vi "EditorThumbnail setLayout.vi"(8 "error in (no error)":errorcluster, 11 "EditorThumbnail in":refnum<class "EditorThumbnail.lvclass">) -> (0 "error out":errorcluster, 3 "EditorThumbnail out":refnum<class "EditorThumbnail.lvclass">)   [LabVIEW 2018, in "EditorThumbnail.lvclass"]
uses:
  EditorThumbnail.lvclass
  <vilib>/Utility/miscctls.llb/LVBoundsTypeDef.ctl
  <vilib>/Utility/miscctls.llb/LVPositionTypeDef.ctl
  EditorThumbnail.lvclass/EditorThumbnail.ctl
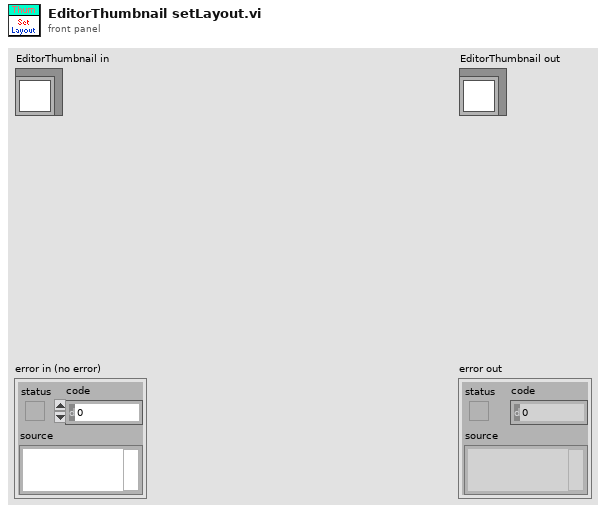
[diagram p1: front panel]
types:
  T1 = typedef "LVPositionTypeDef.ctl" = cluster{"Left":i32, "Top":i32}
  T2 = typedef "LVBoundsTypeDef.ctl" = cluster{"Width":u32, "Height":u32}
  T3 = cluster{"index":u32, "data":cluster{"xdata":dbl[], "ydata":sgl[]}[], "peak":dbl[], "picture":picture}[]
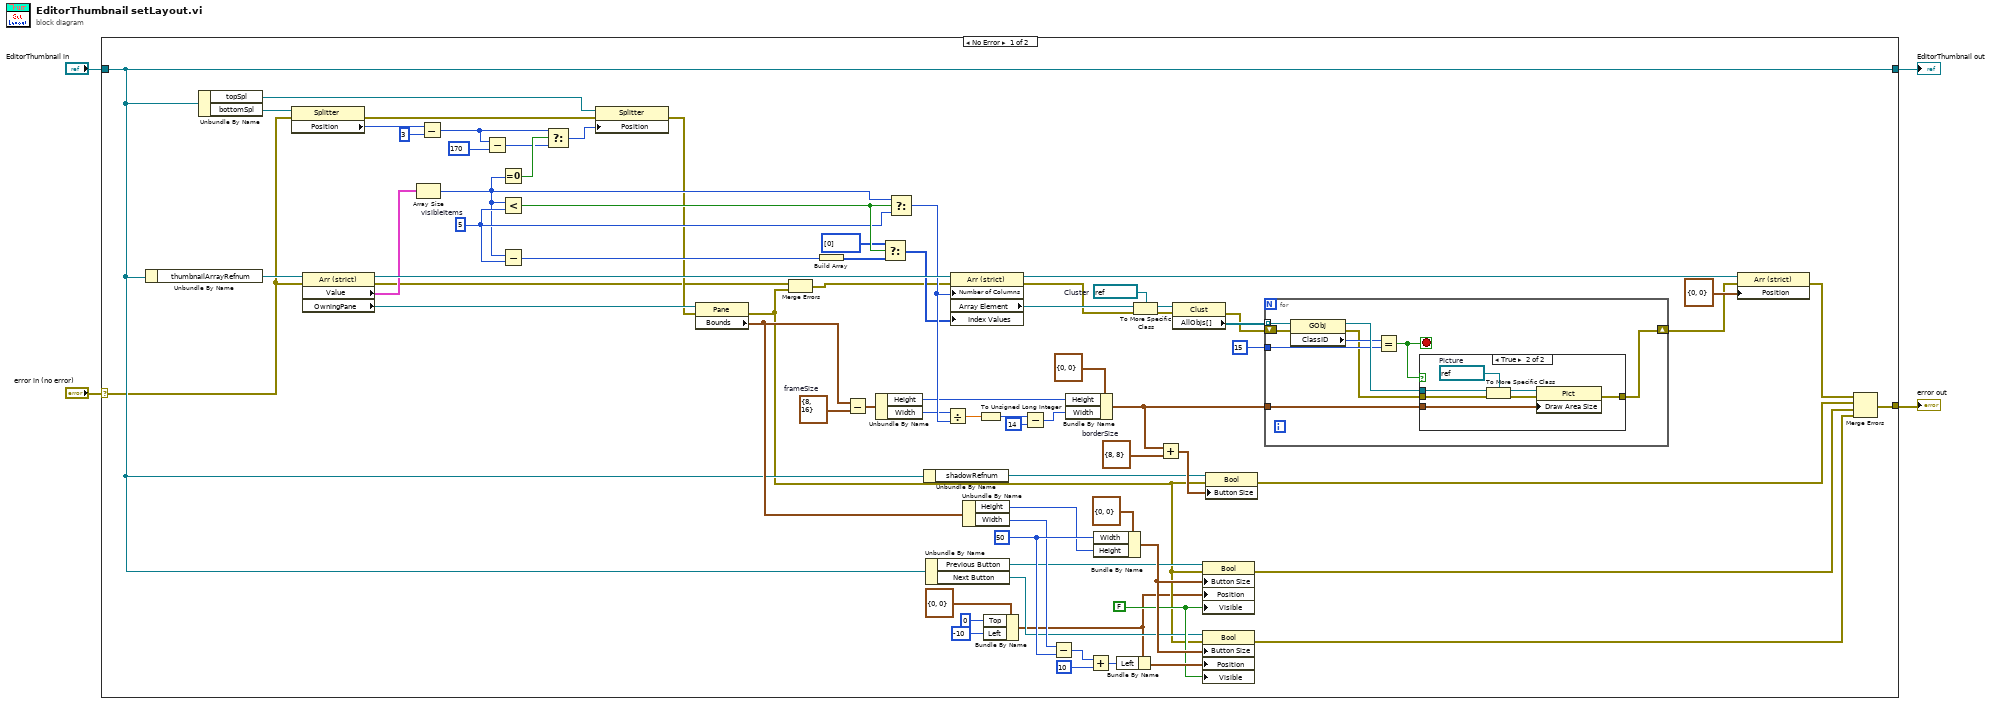
[diagram p0: block diagram]
diagram:
  n1 = case shown="No Error" "error in (no error)" {
    selector: "error in (no error)" -> [w24 w97]
    tunnel: [w49 w97] -> w3
    tunnel: [w26 w96] -> w1
    tunnel: "EditorThumbnail in" -> [w26 w96]
    frame No Error {
      w37 = FALSE ("Visible")
      w40 = u32 50 ("Width")
      w63 = refnum<vi> refnum  # Cluster
      w65 = T2 {"Width"=8, "Height"=8}  # borderSize
      w75 = T2 {"Width"=8, "Height"=16}  # frameSize
      w46 = 5  # visibleItems
      n2 = Unbundle By Name(w26) -> ("thumbnailArrayRefnum"=w78:refnum<vi>)
      n3 = Unbundle By Name(w26) -> ("topSpl"=w15:refnum<vi>, "bottomSpl"=w25:refnum<vi>)
      n4 = property class="Splitter"(reference=w25, error in=w24) -> (error out=w16:errorcluster, "Position"=w21:i32)  [unwired: 1 out]
      n5 = property class="Arr (strict)"(reference=w78, error in=w24) -> (reference out=w76:refnum<vi>, error out=w12:errorcluster, "Value"=w14:T3, "OwningPane"=w77:refnum<vi>)
      n6 = Array Size(array=w14) -> (size(s)=w23:i32)
      n7 = Subtract(x=w21, y=3) -> (x-y=w19:i32)
      n8 = Subtract(x=w19, y=170) -> (x-y=w18:i32)
      n9 = Equal To 0?(x=w23) -> (x = 0?=w20:bool)
      n10 = Less?(x=w23, y=w46) -> (x < y?=w48:bool)
      n11 = Subtract(x=w23, y=w46) -> (x-y=w45:i32)
      n12 = Select(t=w19, s=w20, f=w18) -> (s? t:f=w7:i32)
      n13 = property class="Splitter"(reference=w15, error in=w16, "Position"=w7) -> (error out=w13:errorcluster)  [unwired: 1 out]
      n14 = property class="Pane"(reference=w77, error in=w13) -> (error out=w11:errorcluster, "Bounds"=w36:T2)  [unwired: 1 out]
      n15 = Merge Errors(w12, w11) -> (w10:errorcluster)
      n16 = Build Array(w45) -> (w44:i32[])
      n17 = Subtract(x=w36, y=w75) -> (x-y=w74:T2)
      n18 = Unbundle By Name(w74) -> ("Height"=w68:u32, "Width"=w72:u32)
      n19 = Select(t=u32[] [0] ("Index Values"), s=w48, f=w44) -> (s? t:f=w43:u32[])
      n20 = Select(t=w23, s=w48, f=w46) -> (s? t:f=w73:i32)
      n21 = Unbundle By Name(w26) -> ("shadowRefnum"=w33:refnum<vi>)
      n22 = Unbundle By Name(w26) -> ("Previous Button"=w32:refnum<vi>, "Next Button"=w31:refnum<vi>)
      n23 = Divide(x=w72, y=w73) -> (x/y=w70:dbl)
      n24 = property class="Arr (strict)"(reference=w76, error in=w10, "Number of Columns"=w73, "Index Values"=w43) -> (reference out=w58:refnum<vi>, error out=w56:errorcluster, "Array Element"=w62:refnum<vi>)
      n25 = Unbundle By Name(w36) -> ("Height"=w35:u32, "Width"=w34:u32)
      n26 = To Unsigned Long Integer(number=w70) -> (unsigned 32bit integer=w69:u32)
      n27 = Bundle By Name(cluster=T1 {"Left"=0, "Top"=0} ("Position"), "Top"=0, "Left"=-10) -> (w6:T1)
      n28 = Subtract(x=w69, y=u32 14) -> (x-y=w67:u32)
      n29 = Subtract(x=w34, y=w40) -> (x-y=w38:u32)
      n30 = Bundle By Name(cluster=T2 {"Width"=0, "Height"=0} ("Draw Area Size"), "Height"=w68, "Width"=w67) -> (w59:T2)
      n31 = Add(x=w38, y=u32 10) -> (x+y=w28:u32)
      n32 = Bundle By Name(cluster=T2 {"Width"=0, "Height"=0} ("Button Size"), "Width"=w40, "Height"=w35) -> (w41:T2)
      n33 = Bundle By Name(cluster=w6, "Left"=w28) -> (w39:T1)
      n34 = To More Specific Class(target class=w63, reference=w62, error in=w56) -> (specific class reference=w61:refnum<vi>, error out=w55:errorcluster)
      n35 = Add(x=w59, y=w65) -> (x+y=w64:T2)
      n36 = property class="Clust"(reference=w61, error in=w55) -> (error out=w54:errorcluster, "AllObjs[]"=w60:refnum<vi>[])  [unwired: 1 out]
      n37 = property class="Bool"(reference=w32, error in=w11, "Button Size"=w41, "Position"=w6, "Visible"=w37) -> (error out=w30:errorcluster)  [unwired: 1 out]
      n38 = property class="Bool"(reference=w31, error in=w11, "Button Size"=w41, "Position"=w39, "Visible"=w37) -> (error out=w29:errorcluster)  [unwired: 1 out]
      n39 = property class="Bool"(reference=w33, error in=w11, "Button Size"=w64) -> (error out=w51:errorcluster)  [unwired: 1 out]
      n40 = for {
        tunnel: w60 -> [w87] mode=indexing
        tunnel: w59 -> [w84]
        tunnel: u32 15 ("x") -> [w81]
        shift-right: [w79] -> w52
        shift-left: w54 -> [w83]
        stop <- w86 stop-if-true
        n41 = property class="GObj"(reference=w87, error in=w83) -> (reference out=w85:refnum<vi>, error out=w80:errorcluster, "ClassID"=w82:u32)
        n42 = Equal?(x=w82, y=w81) -> (x = y?=w86:bool)
        n43 = case shown="True" w86 {
          tunnel: w85 -> [_ w94]
          tunnel: w84 -> [_ w91]
          tunnel: w80 -> [w88 w90]
          tunnel: [w88 w89] -> w79
          frame False {
          }
          frame True {
            w95 = refnum<vi> refnum  # Picture
            n44 = To More Specific Class(target class=w95, reference=w94, error in=w90) -> (specific class reference=w93:refnum<vi>, error out=w92:errorcluster)
            n45 = property class="Pict"(reference=w93, error in=w92, "Draw Area Size"=w91) -> (error out=w89:errorcluster)  [unwired: 1 out]
          }
        }
      }
      n46 = property class="Arr (strict)"(reference=w58, error in=w52, "Position"=T1 {"Left"=0, "Top"=0}) -> (error out=w50:errorcluster)  [unwired: 1 out]
      n47 = Merge Errors(w50, w51, w30, w29) -> (w49:errorcluster)
    }
    frame Error {
    }
  }
  "error out" <- w3
  "EditorThumbnail out" <- w1
